vi "GetTagAttributes.vi"(0 "TextIn":string) -> (14 "Tag":string, 15 "Attributes":T3)   [LabVIEW 2020]
uses:
  <resource>/Framework/Providers/Open_GDS/UML/DesignPattern/SubVIs/DesignPatterns_NodeType.ctl
  <resource>/Framework/Providers/Open_GDS/UML/DesignPattern/SubVIs/DesignPatterns_LinkType.ctl
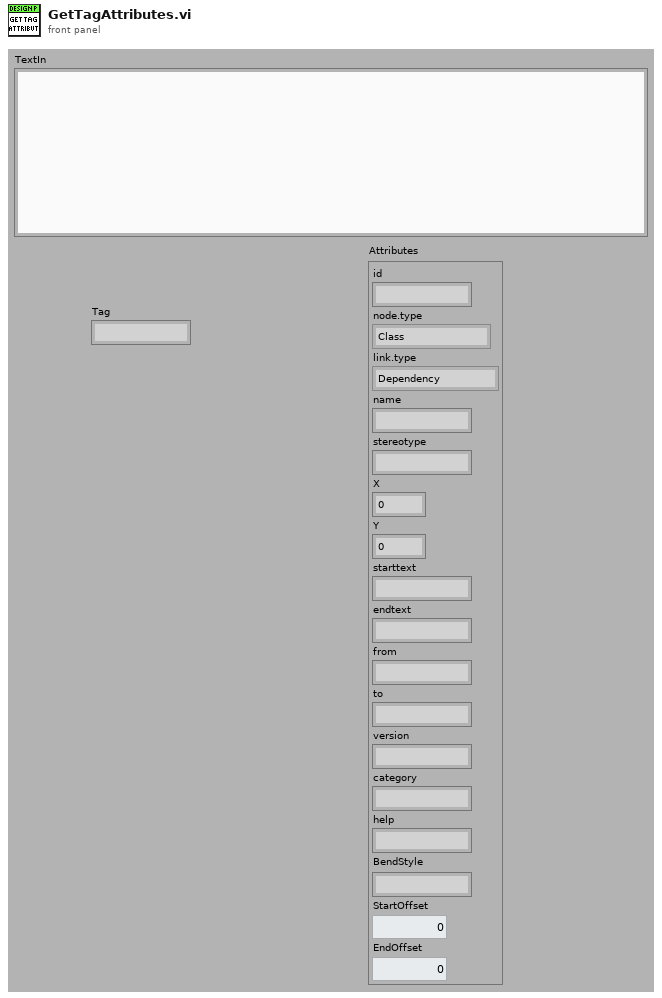
[diagram p1: front panel]
types:
  T1 = typedef "DesignPatterns_NodeType.ctl" = enum16{"Class", "Interface", "Note", "Package"}
  T2 = typedef "DesignPatterns_LinkType.ctl" = enum16{"Dependency", "Inheritance", "Interface", "Association", "Aggregation", "CompositeAggregation"}
  T3 = cluster{"id":string, "node.type":T1, "link.type":T2, "name":string, "stereotype":string, "X":i32, "Y":i32, "starttext":string, "endtext":string, "from":string, "to":string, "version":string, "category":string, "help":string, "BendStyle":string, "StartOffset":i32, "EndOffset":i32}
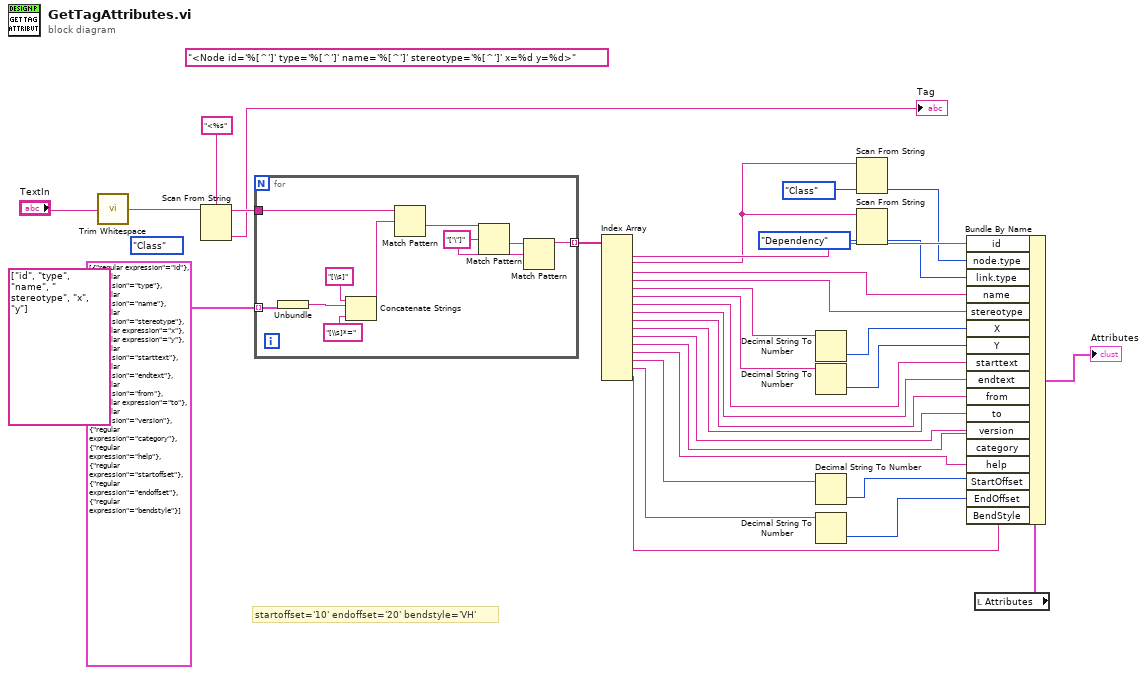
[diagram p0: block diagram]
diagram:
  (unwired) string[] ["id", "type", "name", " stereotype", "x", "y"]
  (unwired) "<Node id='%[^']' type='%[^']' name='%[^']' stereotype='%[^']' x=%d y=%d>" ("format string")
  (unwired) DesignPatterns_NodeType."Class" ("Type")
  # "startoffset='10' endoffset='20' bendstyle='VH'"
  n1 = call <vilib>:"Trim Whitespace.vi"("string"="TextIn") -> ("trimmed string"=w26:string)  [unwired: 1 in]
  n2 = Scan From String(format string="<%s", input string=w26) -> (remaining string=w32:string, output 1=→"Tag":string)  [unwired: 2 in, 3 out]
  n3 = for {
    tunnel: w32 -> [w43]
    tunnel: cluster{"regular expression":string}[] [{"regular expression"="id"}, {"regular expression"="type"}, {"regular expression"="name"}, {"regular expression"="stereotype"}, {"regular expression"="x"}, {"regular expression"="y"}, {"regular expression"="starttext"}, {"regular expression"="endtext"}, {"regular expression"="from"}, {"regular expression"="to"}, {"regular expression"="version"}, {"regular expression"="category"}, {"regular expression"="help"}, {"regular expression"="startoffset"}, {"regular expression"="endoffset"}, {"regular expression"="bendstyle"}] -> [w35] mode=indexing
    tunnel: [w38] -> w30 mode=indexing
    w36 = "['\"]" ("regular expression")
    n4 = Unbundle(w35) -> ("regular expression"=w34:string)
    n5 = Concatenate Strings("[\\s]" ("string"), w34, "[\\s]*=" ("string")) -> (w39:string)
    n6 = Match Pattern(string=w43, regular expression=w39) -> (after substring=w42:string)  [unwired: 4 out]
    n7 = Match Pattern(string=w42, regular expression=w36) -> (after substring=w37:string)  [unwired: 4 out]
    n8 = Match Pattern(string=w37, regular expression=w36) -> (before substring=w38:string)  [unwired: 4 out]
  }
  n9 = Index Array(array=w30) -> (element #1=w24:string, element #2=w19:string, element #3=w17:string, element #4=w16:string, element #5=w29:string, element #6=w28:string, element #7=w13:string, element #8=w12:string, element #9=w11:string, element #10=w10:string, element #11=w8:string, element #12=w7:string, element #13=w6:string, element #14=w4:string, element #15=w2:string, element #16=w5:string)  [unwired: 16 in]
  n10 = Decimal String To Number(string=w29) -> (number=w15:i32)  [unwired: 3 out]
  n11 = Decimal String To Number(string=w28) -> (number=w14:i32)  [unwired: 3 out]
  n12 = Decimal String To Number(string=w4) -> (number=w3:i32)  [unwired: 3 out]
  n13 = Decimal String To Number(string=w2) -> (number=w1:i32)  [unwired: 3 out]
  n14 = Scan From String(input string=w19, default 1=DesignPatterns_NodeType."Class" ("Type")) -> (output 1=w23:T1)  [unwired: 3 in, 3 out]
  n15 = Scan From String(input string=w19, default 1=DesignPatterns_LinkType."Dependency" ("link.type")) -> (output 1=w18:T2)  [unwired: 3 in, 3 out]
  n16 = local read "Attributes"() -> (w25:T3)
  n17 = Bundle By Name(cluster=w25, "id"=w24, "node.type"=w23, "link.type"=w18, "name"=w17, "stereotype"=w16, "X"=w15, "Y"=w14, "starttext"=w13, "endtext"=w12, "from"=w11, "to"=w10, "version"=w8, "category"=w7, "help"=w6, "StartOffset"=w3, "EndOffset"=w1, "BendStyle"=w5) -> (→"Attributes":T3)
